vi "MagSpecCameraSave.vi"(8 "error in (no error)":errorcluster, 9 "async":bool, 10 "Path":path, 11 "MagSpecCamera in":refnum<class "MagSpecCamera.lvclass">) -> (0 "error out":errorcluster, 3 "MagSpecCamera out":refnum<class "MagSpecCamera.lvclass">)   [LabVIEW 2020, in "MagSpecCamera.lvclass"]
uses:
  MagSpecCamera.lvclass
  MagSpecCamera.lvclass/MagSpecCamera.ctl
  <userlib>/_OpenG.lib/file/file.llb/File Exists - Scalar__ogtk.vi
  <vilib>/Utility/file.llb/Write To Spreadsheet File (string).vi
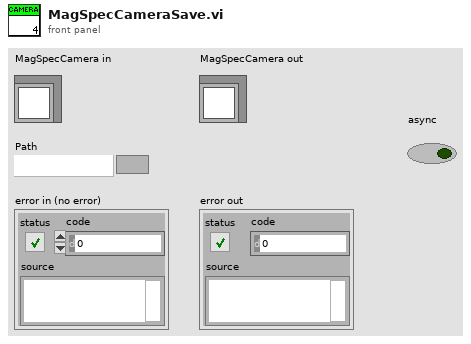
[diagram p1: front panel]
types:
  T1 = typedef "IMAQ Image.ctl" = refnum<image>
  T2 = typedef "OnOffTypeDef.ctl" = enum16{"off", "on"}
  T3 = typedef "Image Type" = u32
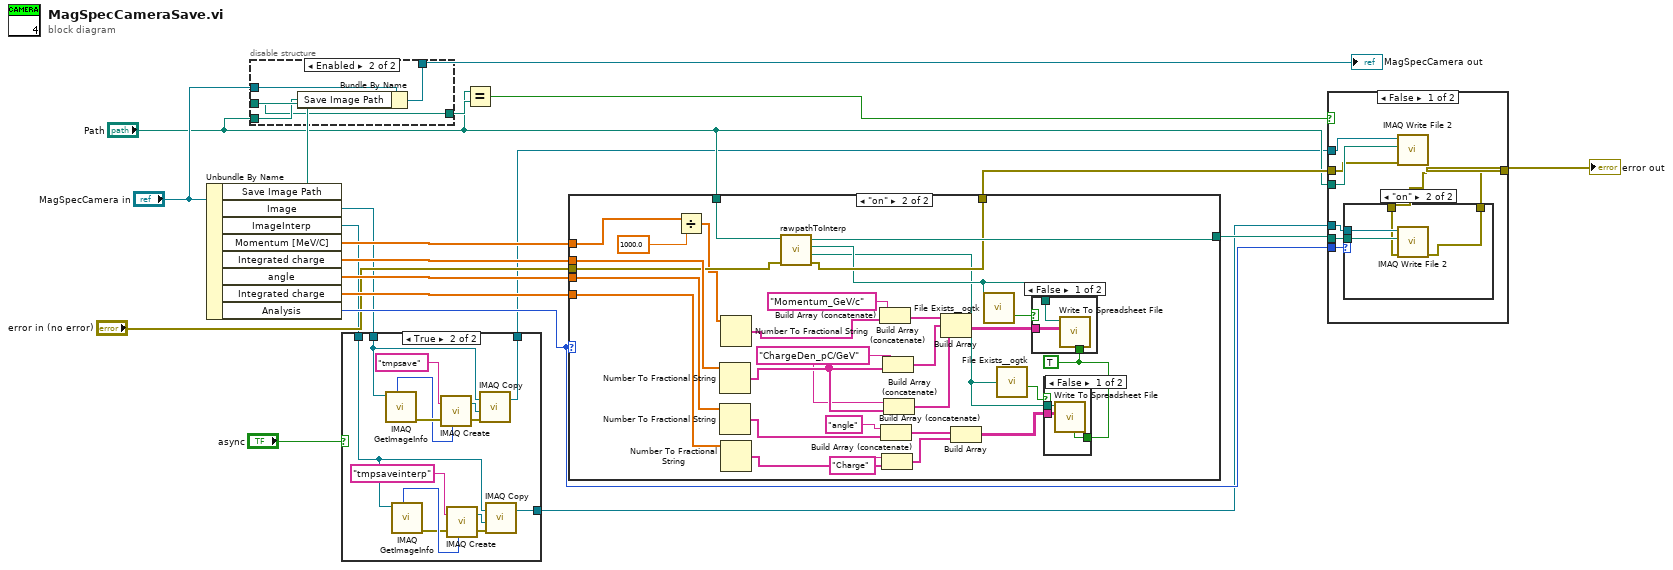
[diagram p0: block diagram]
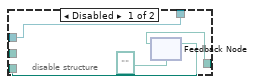
[diagram p6: hidden frame]
diagram:
  n1 = Unbundle By Name("MagSpecCamera in") -> ("Save Image Path"=w12:path, "Image"=w4:T1, "ImageInterp"=w2:T1, "Momentum [MeV/C]"=w13:dbl[], "Integrated charge"=w14:dbl[], "angle"=w18:dbl[], "Integrated charge"=w19:dbl[], "Analysis"=w20:T2)
  n2 = disable-structure shown="Enabled" {
    disable-tunnel: "Path" -> [w23 w27]
    disable-tunnel: [w22 w25] -> w8
    disable-tunnel: "MagSpecCamera in" -> [w21 w28]
    disable-tunnel: [w21 w26] -> w11
    disable-tunnel: w12 -> [_ w25]
    frame Disabled {
      n3 = feedback #1(path "") -> (w22:path)
      n4 = feedback-in #1(w23) -> ()
    }
    frame Enabled {
      n5 = Bundle By Name(cluster=w28, "Save Image Path"=w27) -> (w26:refnum<class "MagSpecCamera.lvclass">)
    }
  }
  "MagSpecCamera out" <- w11
  n6 = case shown="True" "async" {
    tunnel: w4 -> [w30 w34]
    tunnel: [w30 w33] -> w3
    tunnel: w2 -> [w29 w32]
    tunnel: [w29 w31] -> w1
    frame False {
    }
    frame True {
      n7 = call "IMAQ GetImageInfo"("Image"=w34) -> ("error out"=w43:errorcluster, "Image Type"=w41:T3)  [unwired: 3 in, 6 out]
      n8 = call "IMAQ GetImageInfo"("Image"=w32) -> ("error out"=w36:errorcluster, "Image Type"=w38:T3)  [unwired: 3 in, 6 out]
      n9 = call "IMAQ Create"("Image Name"="tmpsave", "Image Type"=w41, "error in (no error)"=w43) -> ("New Image"=w42:T1, "error out"=w44:errorcluster)  [unwired: 2 in]
      n10 = call "IMAQ Create"("Image Name"="tmpsaveinterp", "Image Type"=w38, "error in (no error)"=w36) -> ("New Image"=w37:T1, "error out"=w35:errorcluster)  [unwired: 2 in]
      n11 = call "IMAQ Copy"("error in (no error)"=w44, "Image Dst"=w42, "Image Src"=w34) -> ("Image Dst Out"=w33:T1)  [unwired: 3 in, 1 out]
      n12 = call "IMAQ Copy"("error in (no error)"=w35, "Image Dst"=w37, "Image Src"=w32) -> ("Image Dst Out"=w31:T1)  [unwired: 3 in, 1 out]
    }
  }
  n13 = Equal?(x="Path", y=w8) -> (x = y?=w9:bool)
  n14 = case shown="\"on\"" w20 {
    tunnel: "Path" -> [_ w75]
    tunnel: w13 -> [_ w48]
    tunnel: w14 -> [_ w74]
    tunnel: [_ w65] -> w15
    tunnel: "error in (no error)" -> [w45 w64]
    tunnel: [w45 w63] -> w17
    tunnel: w18 -> [_ w62]
    tunnel: w19 -> [_ w61]
    frame "off", Default {
    }
    frame "on" {
      w53 = TRUE ("transpose? (no:F)")
      w67 = "ChargeDen_pC/GeV" ("format string")
      n15 = Divide(x=w48, y=1000.0 ("Numeric")) -> (x/y=w47:dbl[])
      n16 = Number To Fractional String(number=w74) -> (F-format string=w68:string[])  [unwired: 3 in]
      n17 = Number To Fractional String(number=w62) -> (F-format string=w55:string[])  [unwired: 3 in]
      n18 = Number To Fractional String(number=w47) -> (F-format string=w73:string[])  [unwired: 3 in]
      n19 = Number To Fractional String(number=w61) -> (F-format string=w59:string[])  [unwired: 3 in]
      n20 = call "rawpathToInterp.vi"("error in (no error)"=w64, "Path"=w75) -> ("error out"=w63:errorcluster, "Angle lineout path"=w49:path, "Spectrum lineout path"=w52:path, "Interpolated image path"=w65:path)  [unwired: 6 in]
      n21 = Build Array (concatenate)("Momentum_GeV/c" ("format string"), w73) -> (w71:string[])
      n22 = Build Array (concatenate)("angle" ("format string"), w55) -> (w56:string[])
      n23 = Build Array (concatenate)("Charge" ("format string"), w59) -> (w58:string[])
      n24 = Build Array (concatenate)(w67, w68) -> (w70:string[])
      n25 = Build Array (concatenate)(w67, w68) -> (w66:string[])
      n26 = Build Array(w71, w70, w66) -> (w69:string[][])
      n27 = Build Array(w56, w58) -> (w57:string[][])
      n28 = call-poly <userlib>:"File Exists__ogtk.vi"("file path"=w52) -> ("exists"=w51:bool)  [unwired: 6 in, 1 out]
      n29 = call-poly <userlib>:"File Exists__ogtk.vi"("file path"=w49) -> ("exists"=w50:bool)  [unwired: 6 in, 1 out]
      n30 = case shown="False" w51 {
        tunnel: w69 -> [w81 _]
        tunnel: w53 -> [w80 _]
        tunnel: w52 -> [w79 _]
        frame False {
          n31 = call-poly <vilib>:"Write To Spreadsheet File.vi"("transpose? (no:F)"=w80, "2D data"=w81, "file path (dialog if empty)"=w79) -> ()  [unwired: 5 in, 1 out]
        }
        frame True {
        }
      }
      n32 = case shown="False" w50 {
        tunnel: w57 -> [w78 _]
        tunnel: w49 -> [w77 _]
        tunnel: w53 -> [w76 _]
        frame False {
          n33 = call-poly <vilib>:"Write To Spreadsheet File.vi"("transpose? (no:F)"=w76, "2D data"=w78, "file path (dialog if empty)"=w77) -> ()  [unwired: 5 in, 1 out]
        }
        frame True {
        }
      }
    }
  }
  n34 = case shown="False" w9 {
    tunnel: w3 -> [w87 _]
    tunnel: w17 -> [w88 w95]
    tunnel: [w83 w95] -> w6
    tunnel: "Path" -> [w89 _]
    tunnel: w15 -> [w86 _]
    tunnel: w1 -> [w85 _]
    tunnel: w20 -> [w82 _]
    frame False {
      n35 = call-poly "IMAQ Write File 2"("error in (no error)"=w88, "File Path"=w89, "Image"=w87) -> ("error out"=w84:errorcluster)  [unwired: 7 in, 1 out]
      n36 = case shown="\"on\"" w82 {
        tunnel: w86 -> [_ w94]
        tunnel: w85 -> [_ w93]
        tunnel: w84 -> [w90 w92]
        tunnel: [w90 w91] -> w83
        frame "off", Default {
        }
        frame "on" {
          n37 = call-poly "IMAQ Write File 2"("error in (no error)"=w92, "File Path"=w94, "Image"=w93) -> ("error out"=w91:errorcluster)  [unwired: 7 in, 1 out]
        }
      }
    }
    frame True {
    }
  }
  "error out" <- w6
